vi "creat_dbconn.vi"() -> (0 "错误输出":errorcluster, 3 "连接结果":bool, 8 "错误输入":errorcluster)   [LabVIEW 2015]
uses:
  global/tcp_conn.vi
panel:
  out "response":string
  # "调用本模块，就可自动创建远程数据库连接。"
  # "注：\n1、在labview程序打开的时候创建\n（因为要在程序运行过程中保持连接）"
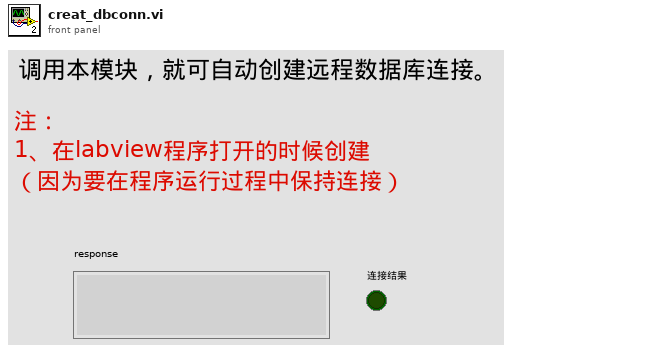
[diagram p1: front panel]
types:
  T1 = enum16{"Standard", "Buffered", "CRLF", "Immediate"}
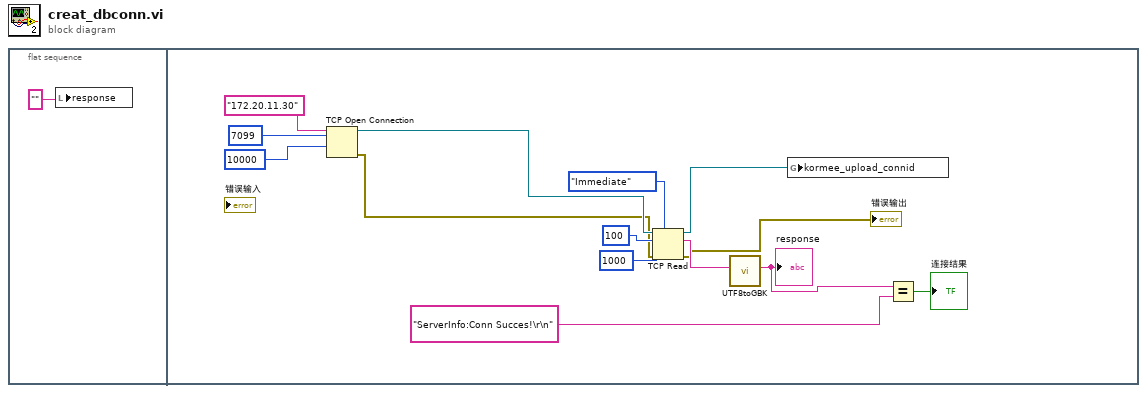
[diagram p0: block diagram]
diagram:
  n1 = flat-sequence {
    frame #0 {
      n2 = local write "response"("" ("response")) -> ()
    }
    frame #1 {
      n3 = TCP Open Connection(address="172.20.11.30" ("地址"), remote port or service name=u16 7099 ("远程端口或服务名称"), timeout ms (60000)=10000 ("超时毫秒(60000)")) -> (connection ID=w9:refnum<k5>, error out=w4:errorcluster)  [unwired: 2 in]
      n4 = TCP Read(connection ID=w9, bytes to read=100 ("读取的字节"), error in (no error)=w4, 7:T1."Immediate" ("模式（标准）"), 9:1000 ("超时毫秒(25000)")) -> (connection ID out=w8:refnum<k5>, data out=w10:string, error out=→"错误输出":errorcluster)
      n5 = call "UTF8toGBK.vi"("UTF-8"=w10) -> ("GBK"=w6:string)  [unwired: 10 in]
      "response" <- w6
      n6 = global write "tcp_conn.vi" "kormee_upload_connid"(w8) -> ()
      n7 = Equal?(x=w6, y="ServerInfo:Conn Succes!\r\n") -> (x = y?=→"连接结果":bool)
    }
  }
